vi "Load App.vi"(8 "Error In":errorcluster, 9 "Open Actor Core front panel? (F)":bool, 10 "Monitor-Pulse.lvclass":refnum<class "Monitor-Pulse.lvclass">, 11 "Status Notifier":refnum<notifier>) -> (0 "Error Out":errorcluster)   [LabVIEW 2015, in "Monitor-Pulse.lvclass"]
uses:
  Monitor-Pulse.lvclass
  Measure Controller/Measure Controller.lvclass/Measure Controller.ctl
  <vilib>/ActorFramework/Actor/Actor.lvclass
  Measure Controller/Measure Controller.lvclass
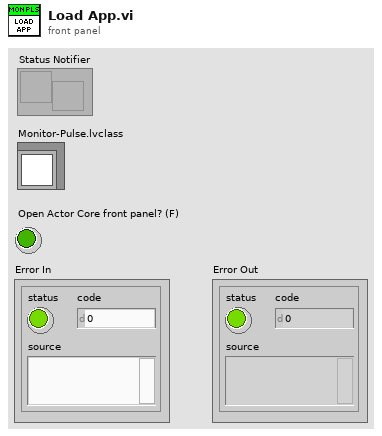
[diagram p1: front panel]
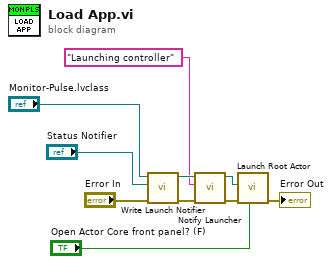
[diagram p0: block diagram]
diagram:
  n1 = call "Write Launch Notifier.vi"("error in (no error)"="Error In", "Launch Notifier"="Status Notifier", "Measure Controller in"="Monitor-Pulse.lvclass") -> ("error out"=w7:errorcluster, "Measure Controller out"=w9:refnum<class "Monitor-Pulse.lvclass">)  [unwired: 7 in]
  n2 = call-dynamic "Notify Launcher.vi"("error in (no error)"=w7, "Notification"="Launching controller" ("notification"), "Measure Controller in"=w9) -> ("error out"=w5:errorcluster, "Measure Controller out"=w6:refnum<class "Monitor-Pulse.lvclass">)  [unwired: 7 in]
  n3 = call <vilib>:"Launch Root Actor.vi"("Open Actor Core front panel? (F)"="Open Actor Core front panel? (F)", "error in (no error)"=w5, "Actor"=w6) -> ("error out"=→"Error Out":errorcluster)  [unwired: 7 in, 1 out]
